vi "Define 2D Wave PDE (Numeric).vi"(0 "PDE in":refnum<class "NI_PDE.lvclass">, 5 "F(t, x, y)":dbl[][][](array[numeric]), 7 "k":dbl=1.0, 9 "a":dbl, 11 "error in (no error)":errorcluster) -> (4 "PDE out":refnum<class "NI_PDE.lvclass">, 15 "error out":errorcluster)   [LabVIEW 2020, in "NI_PDE.lvlib"]
doc: "Defines the right side of a partial differential equation and its coefficients. You must manually select the polymorphic instance to use."
uses:
  <vilib>/gmath/NI_PDE.lvlib
  <vilib>/gmath/pde.llb/PDEClass/NI_PDE.lvclass
  <vilib>/gmath/pde.llb/RHSClass/RHS_3D_Numeric/NI_RHS_3D_Numeric.lvclass
  e:/builds/penguin/labview/branches/2020/dev/dist/vi.lib/gmath/pde.llb/RHSClass/NI_RHS.lvclass
  <vilib>/gmath/pde.llb/PDEClass/PDE_Wave_2D/NI_PDE_Wave_2D.lvclass
  e:/builds/penguin/labview/branches/2020/dev/dist/vi.lib/gmath/pde.llb/PDEClass/NI_PDE.lvclass
  <vilib>/gmath/pde.llb/PDEClass/PDE_2ndOrder_ConstPara/Para Data.ctl
  <vilib>/gmath/pde.llb/PDEClass/PDE_2ndOrder_ConstPara/NI_PDE_2ndOrder_ConstPara.lvclass
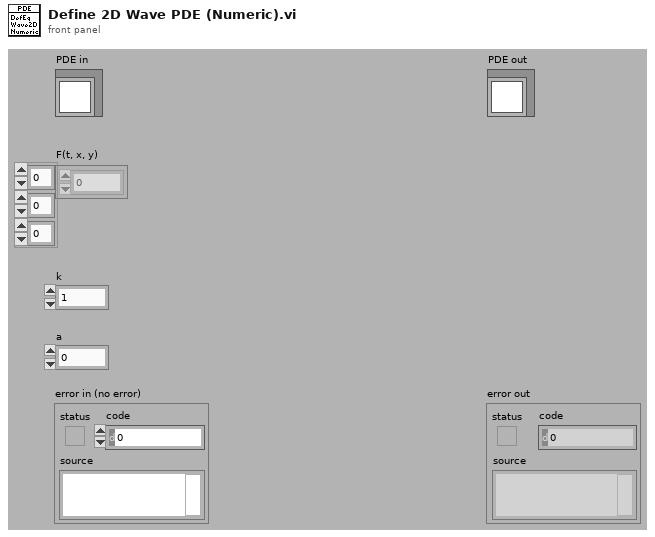
[diagram p1: front panel]
types:
  T1 = typedef "NI_PDE.lvlib/NI_PDE_2ndOrder_ConstPara.lvclass/Para Data.ctl" = cluster{"k":dbl, "a":dbl}
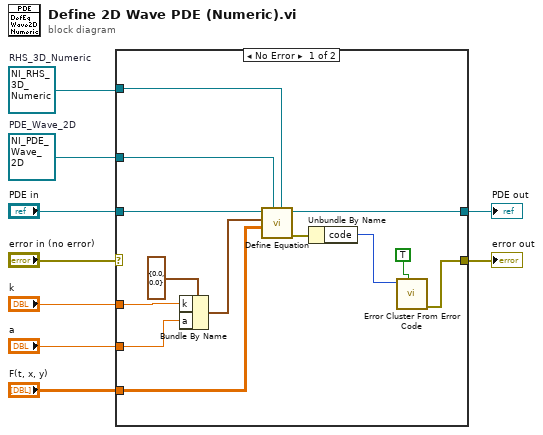
[diagram p0: block diagram]
diagram:
  w1 = refnum<class "NI_PDE_Wave_2D.lvclass"> refnum  # PDE_Wave_2D
  w2 = refnum<class "NI_RHS_3D_Numeric.lvclass"> refnum  # RHS_3D_Numeric
  n1 = case shown="No Error" "error in (no error)" {
    selector: "error in (no error)" -> [_ w24]
    tunnel: "PDE in" -> [w11 w23]
    tunnel: [w17 w23] -> w8
    tunnel: "F(t, x, y)" -> [w14 _]
    tunnel: "a" -> [w13 _]
    tunnel: "k" -> [w15 _]
    tunnel: [w20 w24] -> w3
    tunnel: w1 -> [w12 _]
    tunnel: w2 -> [w10 _]
    frame No Error {
      n2 = Bundle By Name(cluster=T1 {"k"=0.0, "a"=0.0} ("para data"), "k"=w15, "a"=w13) -> (w19:T1)
      n3 = call <vilib>:"Define Equation.vi"("target RHS"=w10, "target PDE"=w12, "RHS"=w14, "parameter"=w19, "PDE in"=w11) -> ("error out"=w16:errorcluster, "PDE out"=w17:refnum<class "NI_PDE.lvclass">)  [unwired: 1 in, 4 out]
      n4 = Unbundle By Name(w16) -> ("code"=w22:i32)
      n5 = call <vilib>:"Error Cluster From Error Code.vi"("show call chain? (False)"=TRUE, "error code (0)"=w22) -> ("error out"=w20:errorcluster)  [unwired: 1 in, 6 out]
    }
    frame Error {
    }
  }
  "PDE out" <- w8
  "error out" <- w3
